vi "Configure Synthesizer Mode.vi"(8 "error in (no error)":errorcluster, 10 "Synthesizer Mode":enum16{"Normal", "Low Noise"}(ring), 11 "PSG-MXG in":refnum<class "PSG-MXG.lvclass">) -> (0 "error out":errorcluster, 3 "PSG-MXG out":refnum<class "PSG-MXG.lvclass">)   [LabVIEW 2020, in "PSG-MXG.lvclass"]
uses:
  PSG-MXG.lvclass
  Signal Generator.lvclass
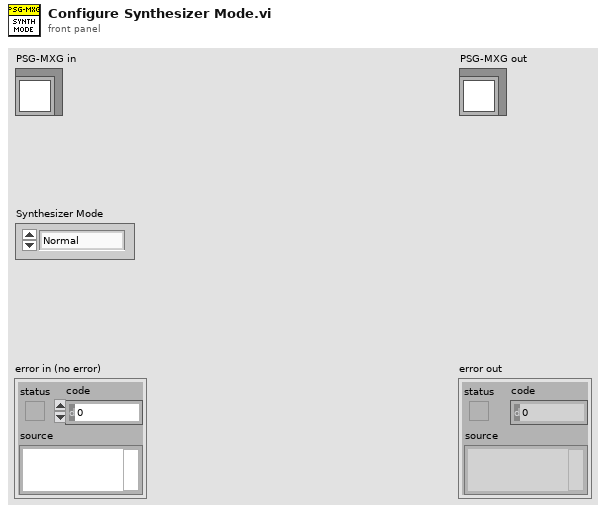
[diagram p1: front panel]
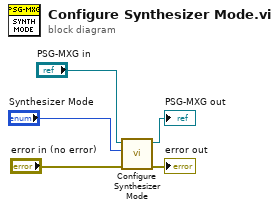
[diagram p0: block diagram]
diagram:
  n1 = call-parent "Configure Synthesizer Mode.vi"("error in (no error)"="error in (no error)", "Synthesizer Mode"="Synthesizer Mode", "Signal Generator in"="PSG-MXG in") -> ("error out"=→"error out":errorcluster, "Signal Generator out"=→"PSG-MXG out":refnum<class "PSG-MXG.lvclass">)  [unwired: 7 in]
